vi "file_name_utils_script.vi"() -> (1 "import statement":string="labVIEW_utils", 3 "file_name_utilities_script":string="labVIEW_utils")   [LabVIEW 2018, in "Python.lvclass"]
uses:
  Python.lvclass
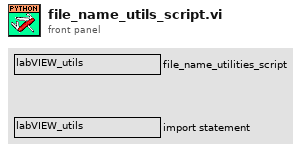
[diagram p1: front panel]
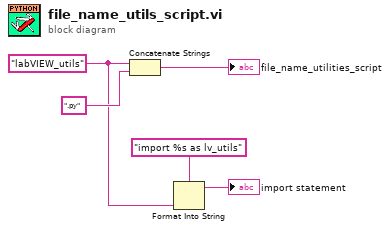
[diagram p0: block diagram]
diagram:
  w2 = "labVIEW_utils" ("name or relative path")
  n1 = Concatenate Strings(w2, ".py" ("string")) -> (→"file_name_utilities_script":string)
  n2 = Format Into String(format string="import %s as lv_utils" ("string"), w2) -> (resulting string=→"import statement":string)  [unwired: 2 in, 1 out]
